vi "(SubVI) Calculate RxnTime for Centering Data_YCC.vi"(4 "sec array":i32[](array[numeric]), 5 "min array":i32[](array[numeric]), 6 "hr array":i32[](array[numeric])) -> (1 "Time past (s)":i32[](array[numeric]))   [LabVIEW 2014]
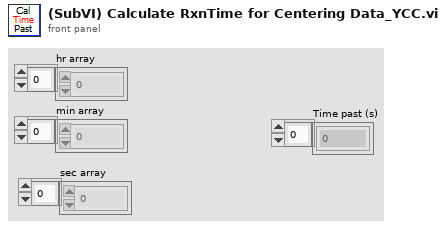
[diagram p1: front panel]
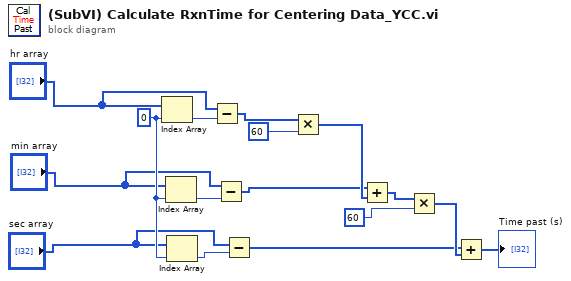
[diagram p0: block diagram]
diagram:
  w14 = 0 ("index")
  n1 = Index Array(array="hr array", index=w14) -> (element=w16:i32)
  n2 = Index Array(array="min array", index=w14) -> (element=w12:i32)
  n3 = Index Array(array="sec array", index=w14) -> (element=w13:i32)
  n4 = Subtract(x="hr array", y=w16) -> (x-y=w9:i32[])
  n5 = Subtract(x="min array", y=w12) -> (x-y=w6:i32[])
  n6 = Subtract(x="sec array", y=w13) -> (x-y=w2:i32[])
  n7 = Multiply(x=w9, y=60 ("hr/min/s")) -> (x*y=w7:i32[])
  n8 = Add(x=w6, y=w7) -> (x+y=w5:i32[])
  n9 = Multiply(x=w5, y=60 ("hr/min/s")) -> (x*y=w3:i32[])
  n10 = Add(x=w2, y=w3) -> (x+y=→"Time past (s)":i32[])
